vi "提取扭矩角度.vi"(11 "字符串":string="B1_011308090450260075.280040.000090.00A000002600000020009999AA ") -> (1 "角度值":string, 3 "扭矩值":string)   [LabVIEW 2013]
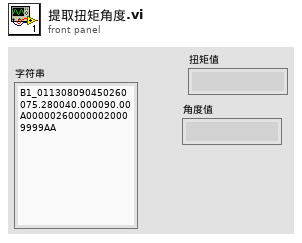
[diagram p1: front panel]
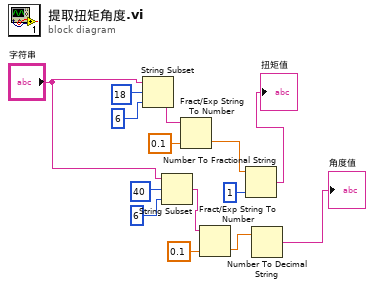
[diagram p0: block diagram]
diagram:
  n1 = String Subset(string="字符串", offset (0)=18 ("偏移量(0)"), length (rest)=6 ("长度（剩余）")) -> (substring=w6:string)
  n2 = String Subset(string="字符串", offset (0)=40 ("偏移量(0)"), length (rest)=6 ("长度（剩余）")) -> (substring=w9:string)
  n3 = Fract/Exp String To Number(string=w6, default (0 dbl)=0.1 ("默认(0 DBL)")) -> (number=w5:dbl)  [unwired: 2 in, 1 out]
  n4 = Fract/Exp String To Number(string=w9, default (0 dbl)=0.1 ("默认(0 DBL)")) -> (number=w7:dbl)  [unwired: 2 in, 1 out]
  n5 = Number To Fractional String(number=w5, precision (6)=i16 1 ("精度(6)")) -> (F-format string=→"扭矩值":string)  [unwired: 2 in]
  n6 = Number To Decimal String(number=w7) -> (decimal integer string=→"角度值":string)  [unwired: 1 in]
